vi "1a_Datalog read.vi"() -> ()   [LabVIEW 2010]
panel:
  out "?":i32
  out "?":dbl[][](graph)
  in  "Cluster":T1
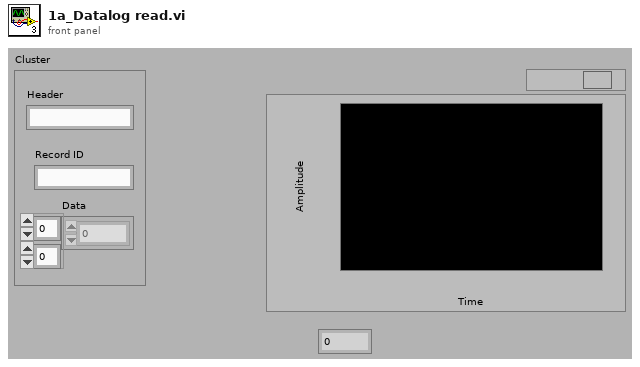
[diagram p1: front panel]
types:
  T1 = cluster{"Data":dbl[][], "Header":string, "Record ID":string}
  T2 = enum16{"open", "replace", "create", "open or create", "replace or create", "replace or create with confirmation"}
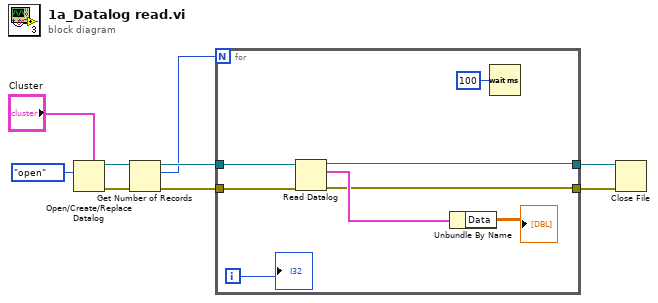
[diagram p0: block diagram]
diagram:
  n1 = Open/Create/Replace Datalog(5:"Cluster", 10:T2."open" ("operation (0:open)")) -> (0:w3:errorcluster, 3:w5:refnum<k1>)  [unwired: 4 in, 1 out]
  n2 = Get Number of Records(4:w3, 7:w5) -> (0:w2:errorcluster, 2:w1:i64, 3:w4:refnum<k1>)
  n3 = for {
    N: w1 -> [_]
    tunnel: w4 -> [w15]
    tunnel: w2 -> [w16]
    tunnel: [w12] -> w8
    tunnel: [w11] -> w7
    i -> [w10]
    n4 = Read Datalog(4:w16, 7:w15) -> (0:w12:errorcluster, 2:w14:T1, 3:w11:refnum<k1>)  [unwired: 1 in]
    n5 = Unbundle By Name(w14) -> ("Data"=→"?":dbl[][])
    n6 = Wait (ms)(milliseconds to wait=u32 100) -> ()  [unwired: 1 out]
    "?" <- w10
  }
  n7 = Close File(refnum=w7, error in=w8) -> ()  [unwired: 2 out]
